vi "match pattern.vi"() -> ()   [LabVIEW 2017]
panel:
  out "offset past match":i32
  out "match substring":string
  out "after substring":string
  out "before substring":string
  in  "String":string
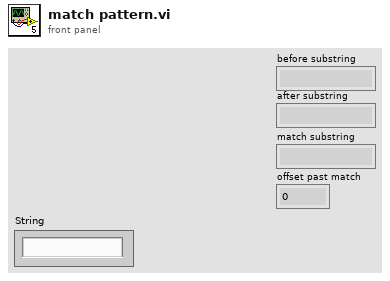
[diagram p1: front panel]
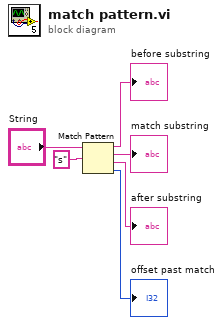
[diagram p0: block diagram]
diagram:
  n1 = Match Pattern(string="String", regular expression="s") -> (before substring=→"before substring":string, match substring=→"match substring":string, after substring=→"after substring":string, offset past match=→"offset past match":i32)  [unwired: 1 in]
